vi "Append List to Report.vi"(0 "report in":refnum<class "NI_HTML.lvclass">, 1 "ordered item type (default)":T1(ring), 2 "unordered item type (default)":enum16{"(default)", "disc", "square", "circle"}(ring), 7 "list elements":string[](array[string]), 9 "list type (ordered)":enum16{"unordered", "ordered"}(ring)=enum."ordered", 11 "error in (no error)":errorcluster, 12 "ordered start (1)":i32=1, 13 "bookmark (Word)":string) -> (4 "report out":refnum<class "NI_HTML.lvclass">, 8 "start out (Word)":i32, 10 "end out (Word)":i32, 15 "error out":errorcluster)   [LabVIEW 2015, in "NI_HTML.lvclass"]
doc: "Adds a list of elements to the report. If you select <B>ordered</B>, the list is numbered or lettered."
uses:
  <vilib>/Utility/NIReport.llb/HTML/NI_HTML.lvclass
  <vilib>/Utility/NIReport.llb/HTML/NI_HTML.lvclass/NI_HTML.ctl
  <vilib>/Utility/NIReport.llb/NI_ReportGenerationCore.lvlib
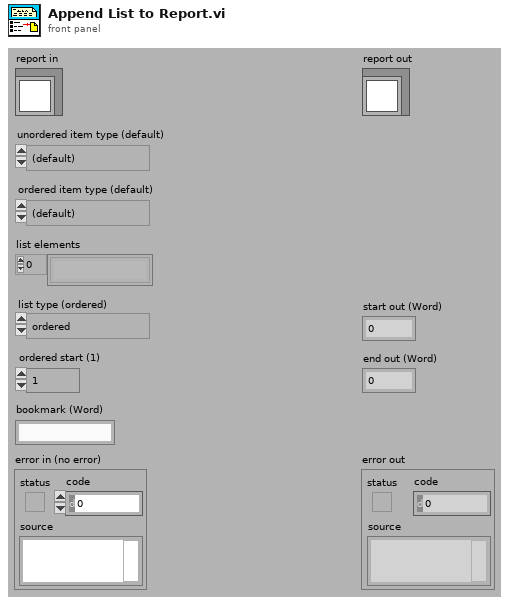
[diagram p1: front panel]
types:
  T1 = enum16{"(default)", "arabic numerals", "lower alpha", "upper alpha"}
  T2 = typedef "NI_ReportGenerationCore.lvlib/HTML Report Data.ctl" = cluster{"Body Text":string, "Font Tag":string, "Title Text":string, "Header Text":string, "Footer Text":string, "Image List":path[]}
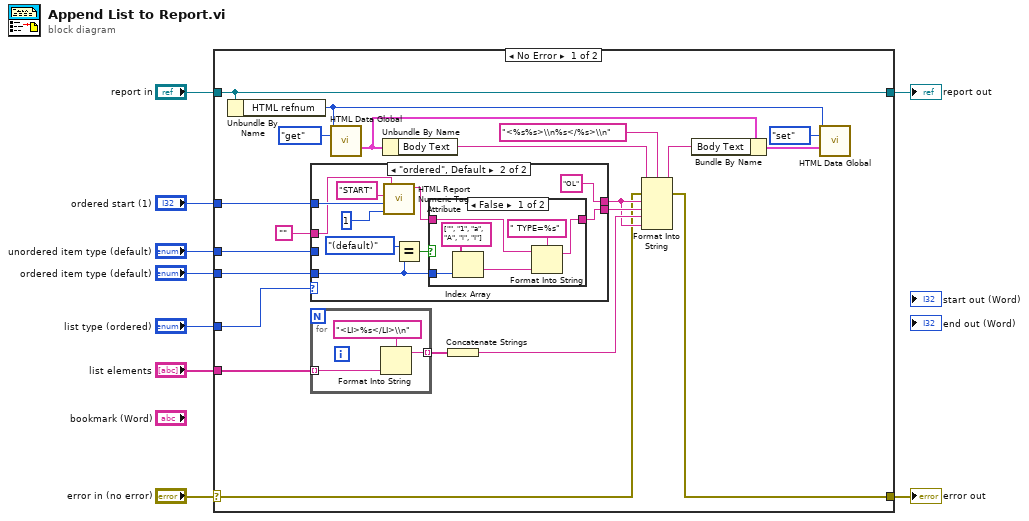
[diagram p0: block diagram]
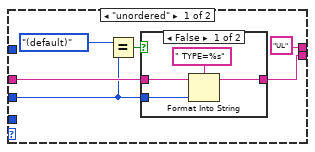
[diagram p2: hidden frame]
diagram:
  n1 = case shown="No Error" "error in (no error)" {
    selector: "error in (no error)" -> [w19 w63]
    tunnel: [w18 w63] -> w8
    tunnel: [w15 w62] -> w6
    tunnel: "report in" -> [w15 w62]
    tunnel: "list elements" -> [w24 _]
    tunnel: "list type (ordered)" -> [w23 _]
    tunnel: "ordered item type (default)" -> [w22 _]
    tunnel: "unordered item type (default)" -> [w21 _]
    tunnel: "ordered start (1)" -> [w20 _]
    frame No Error {
      n2 = Unbundle By Name(w15) -> ("HTML refnum"=w10:u32)
      n3 = case shown="\"ordered\", Default" w23 {
        tunnel: [w35 w48] -> w27
        tunnel: ["UL" "OL"] -> w26
        tunnel: w20 -> [_ w51]
        tunnel: w22 -> [_ w43]
        tunnel: "" -> [w32 w44]
        tunnel: w21 -> [w31 _]
        frame "unordered" {
          n4 = Equal?(x=enum16{"(default)", "disc", "square", "circle"}."(default)" ("y"), y=w31) -> (x = y?=w36:bool)
          n5 = case shown="False" w36 {
            tunnel: w31 -> [w39 _]
            tunnel: [w38 w41] -> w35
            tunnel: w32 -> [w37 w41]
            frame False {
              n6 = Format Into String(format string=" TYPE=%s", initial string=w37, w39) -> (resulting string=w38:string)  [unwired: 1 in, 1 out]
            }
            frame True {
            }
          }
        }
        frame "ordered", Default {
          n7 = call <vilib>:"HTML Report Numeric Tag Attribute.vi"("default value (0)"=1, "value"=w51, "label"="START", "tag attributes in"=w44) -> ("tag attributes out"=w47:string)  [unwired: 3 out]
          n8 = Equal?(x=T1."(default)" ("y"), y=w43) -> (x = y?=w49:bool)
          n9 = case shown="False" w49 {
            tunnel: w43 -> [w54 _]
            tunnel: w47 -> [w56 w58]
            tunnel: [w55 w58] -> w48
            frame False {
              n10 = Index Array(array=string[] ["", "1", "a", "A", "i", "I"] ("labels"), index=w54) -> (element=w53:string)
              n11 = Format Into String(format string=" TYPE=%s", initial string=w56, w53) -> (resulting string=w55:string)  [unwired: 1 in, 1 out]
            }
            frame True {
            }
          }
        }
      }
      n12 = for {
        tunnel: w24 -> [w60] mode=indexing
        tunnel: [w59] -> w28 mode=indexing
        n13 = Format Into String(format string="<LI>%s</LI>\\n", w60) -> (resulting string=w59:string)  [unwired: 2 in, 1 out]
      }
      n14 = call <vilib>:"HTML Data Global.vi"("HTML refnum"=w10, "menu"=enum16{"init", "get", "set", "delete"}."get") -> ("HTML report data out"=w11:T2)  [unwired: 1 in, 12 out]
      n15 = Unbundle By Name(w11) -> ("Body Text"=w16:string)
      n16 = Concatenate Strings(w28) -> (w29:string)
      n17 = Format Into String(format string="<%s%s>\\n%s</%s>\\n", initial string=w16, error in=w19, w26, w27, w29, w26) -> (resulting string=w12:string, error out=w18:errorcluster)
      n18 = Bundle By Name(cluster=w11, "Body Text"=w12) -> (w14:T2)
      n19 = call <vilib>:"HTML Data Global.vi"("HTML refnum"=w10, "menu"=enum16{"init", "get", "set", "delete"}."set", "HTML report data in"=w14) -> ()  [unwired: 13 out]
    }
    frame Error {
    }
  }
  "error out" <- w8
  "report out" <- w6
